vi "SetEntryWaveVoltageLow.vi"(1 "Voltage Low Options":u16(ring) items=["Voltage Low Value", "Default", "Minimum", "Maximum"], 2 "Element":i16=1 min=1, 4 "error in (no error)":errorcluster, 5 "Voltage Low (V)":dbl, 6 "Channel":u16(ring) items=["Channel 1", "Channel 2", "Channel 3", "Channel 4", "Channel 5", "Channel 6", "Channel 7", "Channel 8"], 7 "VISA resource name":refnum<visa-resource-name>) -> (0 "error out":errorcluster, 3 "VISA resource name out":refnum<visa-resource-name>)   [LabVIEW 2020, in "Active Technologies AWG3000.lvlib"]
uses:
  Active Technologies AWG3000.lvlib
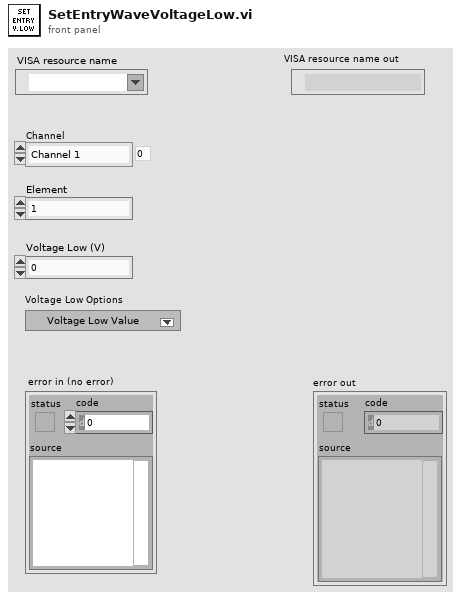
[diagram p1: front panel]
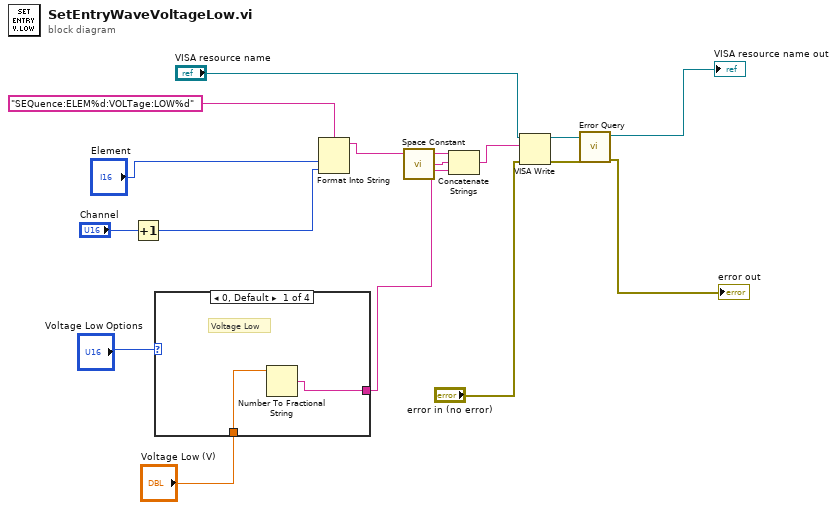
[diagram p0: block diagram]
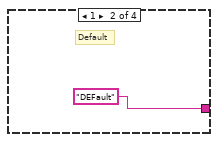
[diagram p2: hidden frame]
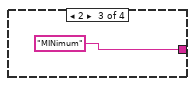
[diagram p3: hidden frame]
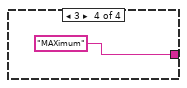
[diagram p4: hidden frame]
diagram:
  n1 = Increment(x="Channel") -> (x+1=w7:u16)
  n2 = case shown="0, Default" "Voltage Low Options" {
    tunnel: [w17 "DEFault" ("write buffer") "MINimum" ("write buffer") "MAXimum" ("write buffer")] -> w2
    tunnel: "Voltage Low (V)" -> [w18 _ _ _]
    frame 0, Default {
      # "Voltage Low"
      n3 = Number To Fractional String(number=w18) -> (F-format string=w17:string)  [unwired: 3 in]
    }
    frame 1 {
      # "Default"
    }
    frame 2 {
    }
    frame 3 {
    }
  }
  n4 = Format Into String(format string="SEQuence:ELEM%d:VOLTage:LOW%d" ("write buffer"), "Element", w7) -> (resulting string=w3:string)  [unwired: 2 in, 1 out]
  n5 = call <vilib>:"Space Constant.vi"() -> ("String"=w4:string)
  n6 = Concatenate Strings(w3, w4, w2) -> (w1:string)
  n7 = VISA Write(VISA resource name="VISA resource name", write buffer=w1, error in (no error)="error in (no error)") -> (VISA resource name out=w13:refnum<visa-resource-name>, error out=w12:errorcluster)  [unwired: 1 out]
  n8 = call "Error Query.vi"("error in (no error)"=w12, "VISA resource name"=w13) -> ("error out"=→"error out":errorcluster, "VISA resource name out"=→"VISA resource name out":refnum<visa-resource-name>)  [unwired: 6 in, 2 out]
